vi "GaGe_TrigConfig.vi"(4 "Trigger":T2 {"Slope" items=["Positive", "Negative"]; "Level" format="%.2f"; "Coupling" items=["DC 1 MOhm", "AC 1 MOhm", "HF Reject", "LF Reject", "AC Plus HF Reject"]; "Source" items=["Chan 1", "External"]}, 5 "Handle Cluster":T1) -> (2 "Handle Cluster Out":T1)   [LabVIEW 2022 SP3]
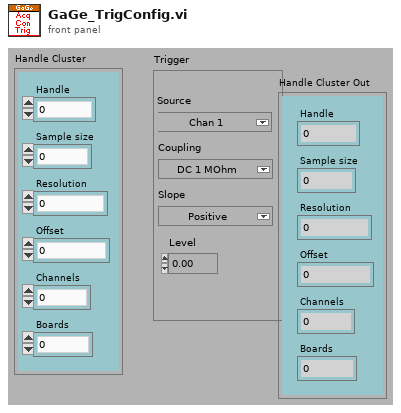
[diagram p1: front panel]
types:
  T1 = cluster{"Handle":u32, "Sample size":u32, "Resolution":i32, "Offset":i32, "Channels":u32, "Boards":u32}
  T2 = cluster{"Source":u16, "Coupling":u16, "Slope":u16, "Level":dbl}
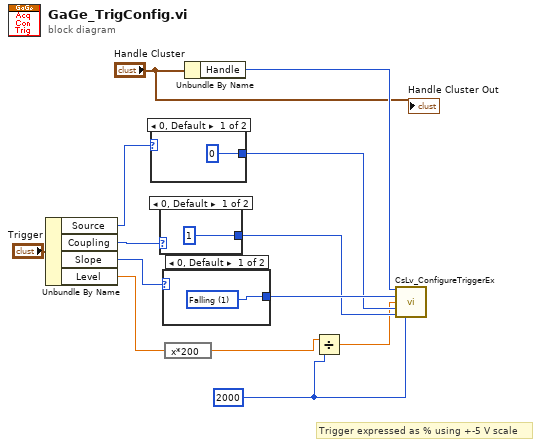
[diagram p0: block diagram]
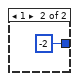
[diagram p2: hidden frame]
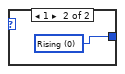
[diagram p3: hidden frame]
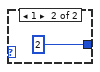
[diagram p4: hidden frame]
diagram:
  w2 = u32 2000 ("External Range (2000 mV)")
  # "Trigger expressed as % using +-5 V scale"
  n1 = Unbundle By Name("Trigger") -> ("Source"=w9:u16, "Coupling"=w12:u16, "Slope"=w11:u16, "Level"=w6:dbl)
  n2 = case shown="0, Default" w9 {
    tunnel: [0 -2] -> w8
    frame 0, Default {
    }
    frame 1 {
    }
  }
  n3 = case shown="0, Default" w12 {
    tunnel: [1 2] -> w7
    frame 0, Default {
    }
    frame 1 {
    }
  }
  n4 = case shown="0, Default" w11 {
    tunnel: [w18 w19] -> w10
    frame 0, Default {
      w18 = 1 items=["Falling"=1, "Negative"=0] ("Triggering:Trigger Slope")
    }
    frame 1 {
      w19 = 0 items=["Positive"=1, "Rising"=0] ("Triggering:Trigger Slope")
    }
  }
  n5 = expression code="x*200"(w6) -> (w3:dbl)
  n6 = Unbundle By Name("Handle Cluster") -> ("Handle"=w5:u32)
  n7 = Divide(x=w3, y=w2) -> (x/y=w4:dbl)
  n8 = call <userlib>:"CsLv_ConfigureTriggerEx.vi"("Handle"=w5, "Slope (1)"=w10, "Level (0)"=w4, "Source (0)"=w8, "Ext. Coupling (1)"=w7, "External Range (2000 mV)"=w2) -> ()  [unwired: 9 in, 1 out]
  "Handle Cluster Out" <- "Handle Cluster"
